vi "Pre-Init.vi"(8 "error in (no error)":errorcluster, 11 "DAQmx Lockin Digitizer Driver in":refnum<class "DAQmx Lockin Digitizer Driver.lvclass">) -> (0 "error out":errorcluster, 3 "DAQmx Lockin Digitizer Driver out":refnum<class "DAQmx Lockin Digitizer Driver.lvclass">)   [LabVIEW 2021, in "DAQmx Lockin Digitizer Driver.lvclass"]
uses:
  DAQmx Lockin Digitizer Driver.lvclass
  C:/GitHub/NHMFL_Core/Libraries/NI-DAQ/DAQmx Digitizer/DAQmx Digitizer.lvclass
  C:/GitHub/NHMFL_Core/Libraries/Instruments/Pulse Driver/Lockin Digitizer Driver/Lockin Digitizer Driver.lvclass
  C:/GitHub/NHMFL_Core/Libraries/Instruments/Pulse Driver/Pulse Driver.lvclass
  DAQmx Digitizer/DAQmx Digitizer.lvclass/DAQmx Digitizer.ctl
  DAQmx Lockin Digitizer Driver.lvclass/DAQmx Lockin Digitizer Driver.ctl
  Instruments/Pulse Driver/Pulse Driver.lvclass/Pulse Driver.ctl
  e6abacbe-9961-4925-8f20-701274b45e77.vi
  DAQmx Digitizer/Read DAQmx Device Name.vi
  Instruments/Pulse Driver/Write Samples per read.vi
  DAQmx Lockin Driver/DAQmx Lockin Driver.lvclass
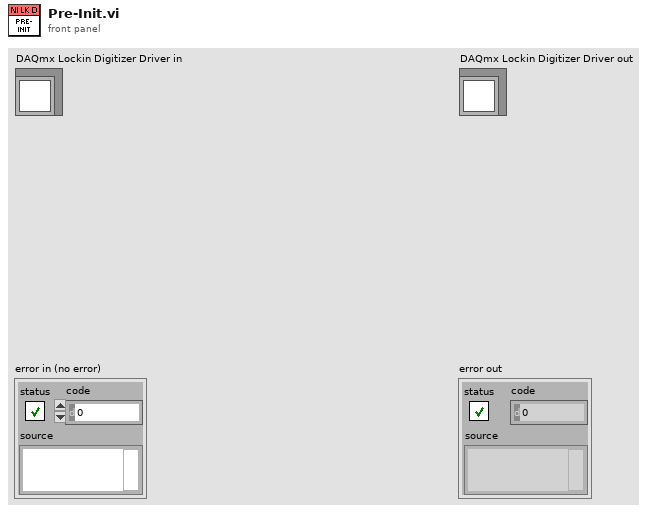
[diagram p1: front panel]
types:
  T1 = typedef "Lockin Digitizer Configuration.ctl" = cluster{"Post-trigger delay":dbl, "Post-trigger duration":dbl, "Rate":dbl, "Ranges":dbl[], "Re-name channels":string[], "Active channels":string, "External\nclock":bool, "Frequencies":dbl[], "Time\nconstant":dbl, "Output \namplitudes":dbl[], "Input\nchannles":string[]}
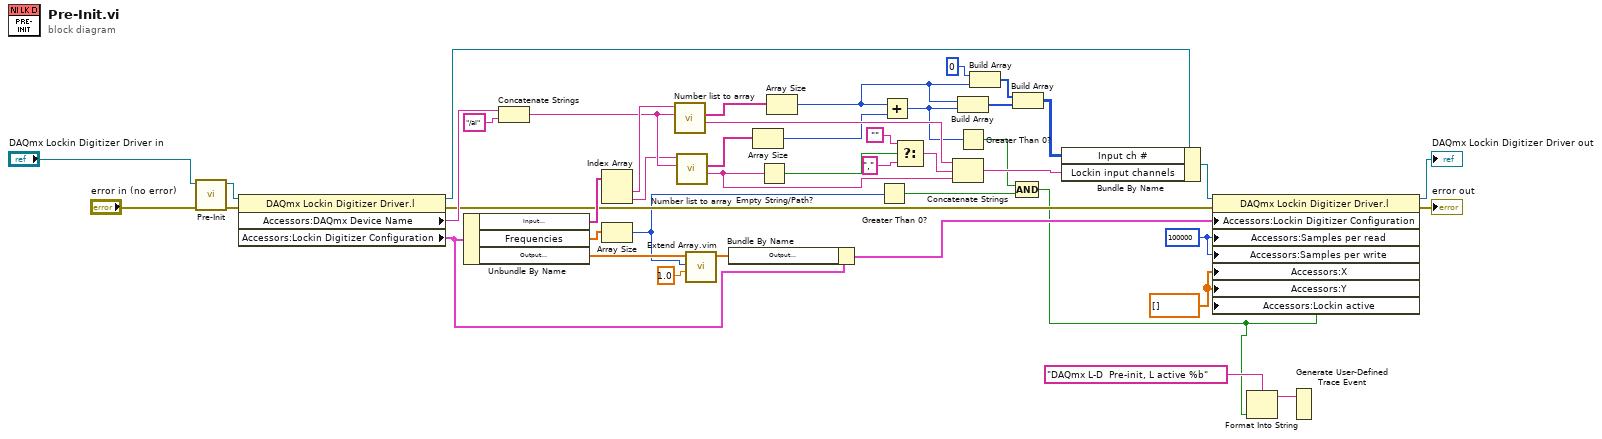
[diagram p0: block diagram]
diagram:
  w5 = dbl[] [] ("X")
  w7 = 100000
  n1 = call-parent "Pre-Init.vi"("error in (no error)"="error in (no error)", "Lockin Digitizer Driver in"="DAQmx Lockin Digitizer Driver in") -> ("error out"=w45:errorcluster, "Lockin Digitizer Driver out"=w42:refnum<class "DAQmx Lockin Digitizer Driver.lvclass">)  [unwired: 8 in]
  n2 = property class="DAQmx Lockin Digitizer Driver.l"(reference=w42, error in=w45) -> (reference out=w21:refnum<class "DAQmx Lockin Digitizer Driver.lvclass">, error out=w10:errorcluster, "Accessors:DAQmx Device Name"=w39:tag, "Accessors:Lockin Digitizer Configuration"=w16:T1)
  n3 = Unbundle By Name(w16) -> ("Input\nchannles"=w41:string[], "Frequencies"=w19:dbl[], "Output \namplitudes"=w18:dbl[])
  n4 = Concatenate Strings(w39, "/ai" ("string")) -> (w37:string)
  n5 = Index Array(array=w41) -> (element #1=w38:string, element #2=w36:string)  [unwired: 2 in]
  n6 = Array Size(array=w19) -> (size(s)=w4:i32)
  n7 = call "Number list to array.vi"("Full names prefix"=w37, "Number list"=w38) -> ("Comma-separated list"=w31:string, "Full names"=w29:string[])  [unwired: 7 in, 1 out]
  n8 = call "Number list to array.vi"("Full names prefix"=w37, "Number list"=w36) -> ("Comma-separated list"=w30:string, "Full names"=w28:string[])  [unwired: 7 in, 1 out]
  n9 = call "Extend Array.vim"("Default value"=1.0, "Extend to size"=w4, "Array in"=w18) -> ("Array out"=w15:dbl[])  [unwired: 7 in, 1 out]
  n10 = Bundle By Name(cluster=w16, "Output \namplitudes"=w15) -> (w8:T1)
  n11 = Array Size(array=w28) -> (size(s)=w23:i32)
  n12 = Empty String/Path?(string/path=w30) -> (empty?=w32:bool)
  n13 = Array Size(array=w29) -> (size(s)=w24:i32)
  n14 = Greater Than 0?(x=w4) -> (x > 0?=w12:bool)
  n15 = Add(x=w24, y=w23) -> (x+y=w6:i32)
  n16 = Select(t="", s=w32, f=",") -> (s? t:f=w35:string)
  n17 = Concatenate Strings(w31, w35, w30) -> (w20:string)
  n18 = Build Array(w24, w6) -> (w27:i32[])
  n19 = Greater Than 0?(x=w6) -> (x > 0?=w13:bool)
  n20 = Build Array(0, w24) -> (w26:i32[])
  n21 = Build Array(w26, w27) -> (w22:i32[][])
  n22 = Compound Arithmetic op=AND(w13, w12) -> (w1:bool)
  n23 = Bundle By Name(cluster=w21, "Input ch #"=w22, "Lockin input channels"=w20) -> (w14:refnum<class "DAQmx Lockin Digitizer Driver.lvclass">)
  n24 = property class="DAQmx Lockin Digitizer Driver.l"(reference=w14, error in=w10, "Accessors:Lockin Digitizer Configuration"=w8, "Accessors:Samples per read"=w7, "Accessors:Samples per write"=w7, "Accessors:X"=w5, "Accessors:Y"=w5, "Accessors:Lockin active"=w1) -> (reference out=→"DAQmx Lockin Digitizer Driver out":refnum<class "DAQmx Lockin Digitizer Driver.lvclass">, error out=→"error out":errorcluster)
  n25 = Format Into String(format string="DAQmx L-D  Pre-init, L active %b" ("string"), w1) -> (resulting string=w3:string)  [unwired: 2 in, 1 out]
  n26 = Generate User-Defined Trace Event(2:w3) -> ()  [unwired: 1 in]
